vi "Last Code Point.vi"(11 "String":string) -> (3 "Last Code Point":string)   [LabVIEW 2020, in "Stream.lvlib" / "URLPattern.lvclass"]
uses:
  URLPattern.lvclass
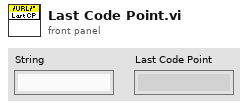
[diagram p1: front panel]
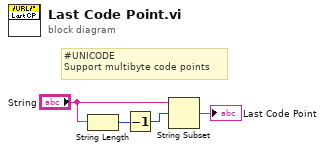
[diagram p0: block diagram]
diagram:
  # "#UNICODE\nSupport multibyte code points"
  n1 = String Length(string="String") -> (length=w4:i32)
  n2 = Decrement(x=w4) -> (x-1=w2:i32)
  n3 = String Subset(string="String", offset (0)=w2) -> (substring=→"Last Code Point":string)  [unwired: 1 in]
